vi "SeriellRead-15-07-17.vi"(6 "SkalierungsfaktorHorst":dbl[](array[numeric]), 7 "VorwortHorst":string[](array[string]), 8 "error in":errorcluster, 9 "Zwischenspeicher":string[](array[string]), 10 "Senden?":bool[](array[boolean]), 11 "FPGA VI Reference In":refnum<k20>) -> (1 "Senden?":bool[](array[boolean]), 2 "Zwischenspeicher":string[](array[string]), 3 "error out":errorcluster)   [LabVIEW 2017]
uses:
  GVECDs.vi
  <vilib>/rvi/interface/nirviMethod/nirviMethod.xnode
  FPGA Bitfiles/HAGAR-V_FPGATarget_FPGA-Programm-05_gdVwCsZS6sg.lvbitx
  FPGA/FPGA-Programm-05-17.vi
  <vilib>/FPGAPlugInAG/cRIO-9114/niLvFpga_ReadFifo_cRIO-9114.vi
  <vilib>/rvi/errors/niLvFpgaMergeErrorWithErrorCode.vi
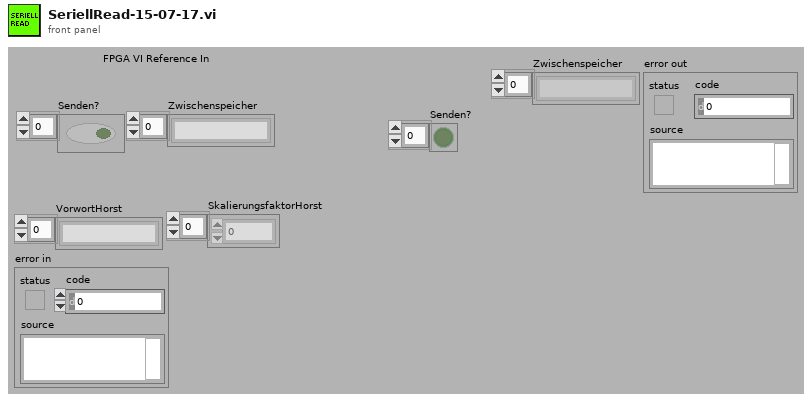
[diagram p1: front panel]
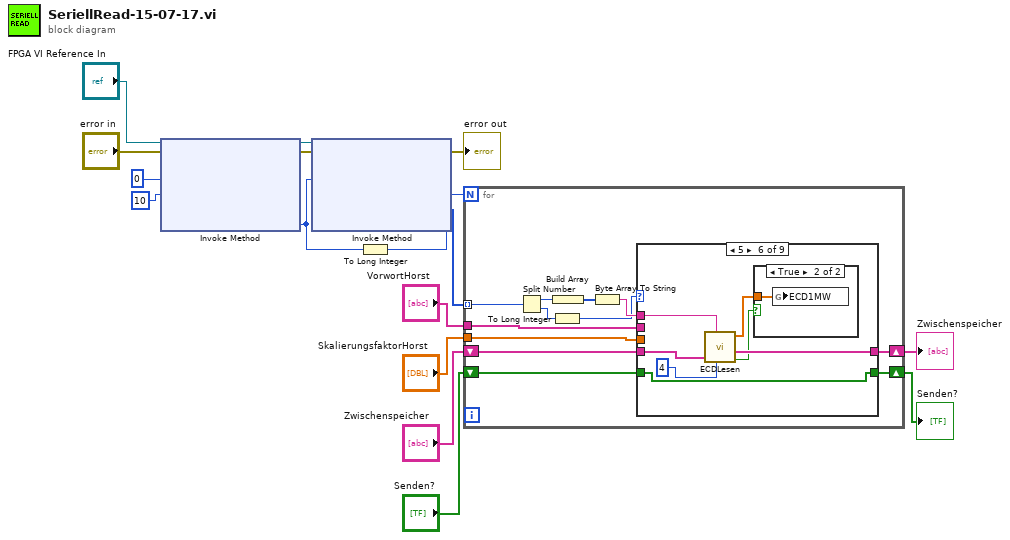
[diagram p0: block diagram]
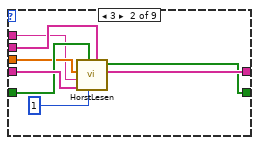
[diagram p3: hidden frame]
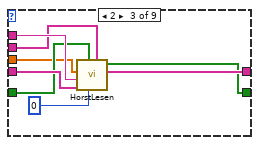
[diagram p4: hidden frame]
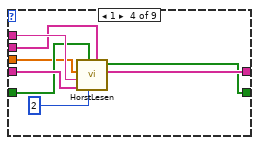
[diagram p5: hidden frame]
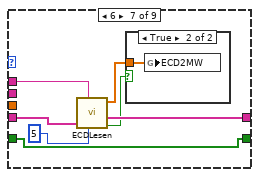
[diagram p8: hidden frame]
diagram:
  n1 = xnode "Invoke Method"("FPGA-VI-Referenz (Eingang)"="FPGA VI Reference In", "Fehler (Eingang)"="error in", "Anzahl der Elemente"=u32 0 ("Number of Elements"), "Timeout (ms)"=10) -> ("FPGA-VI-Referenz (Ausgang)"=w12:refnum<k20>, "Fehler (Ausgang)"=w3:errorcluster, "Verbleibende Elemente"=w15:u32)  [unwired: 1 out]
  n2 = xnode "Invoke Method"("FPGA-VI-Referenz (Eingang)"=w12, "Fehler (Eingang)"=w3, "Anzahl der Elemente"=w15) -> ("Fehler (Ausgang)"=→"error out":errorcluster, "Daten"=w11:u16[])  [unwired: 1 in, 2 out]
  n3 = To Long Integer(number=w15) -> (32bit integer=w16:i32)
  n4 = for {
    N: w16 -> [_]
    tunnel: w11 -> [w28] mode=indexing
    shift-right: [w24] -> w8
    shift-left: "Senden?" -> [w23]
    shift-right: [w25] -> w7
    shift-left: "Zwischenspeicher" -> [w26]
    tunnel: "VorwortHorst" -> [w19]
    tunnel: "SkalierungsfaktorHorst" -> [w18]
    n5 = Split Number(x=w28) -> (hi(x)=w22:u8, lo(x)=w20:u8)
    n6 = To Long Integer(number=w20) -> (32bit integer=w17:i32)
    n7 = Build Array(w22) -> (w21:u8[])
    n8 = Byte Array To String(unsigned byte array=w21) -> (string=w27:string)
    n9 = case shown="5" w17 {
      tunnel: w27 -> [_ w31 w46 w54 _ w63 w71 _ _]
      tunnel: w26 -> [w30 w38 w45 w53 w56 w62 w70 w73 w75]
      tunnel: [w30 w37 w44 w52 w56 w61 w69 w73 w75] -> w25
      tunnel: [w29 w36 w43 w51 w55 w57 w65 w74 w76] -> w24
      tunnel: w23 -> [w29 w35 w42 w50 w55 w57 w65 w74 w76]
      tunnel: w19 -> [_ w34 w41 w49 _ _ _ _ _]
      tunnel: w18 -> [_ w33 w40 w48 _ _ _ _ _]
      frame 0, Default {
      }
      frame 3 {
        n10 = call "HorstLesen.vi"("VorwortHorst"=w34, "Port"=1, "Senden?"=w35, "Zwischenspeicher"=w38, "string"=w31, "SkalierungsfaktorHorst"=w33) -> ("Zwischenspeicher"=w37:string[], "Senden?"=w36:bool[])  [unwired: 4 in]
      }
      frame 2 {
        n11 = call "HorstLesen.vi"("VorwortHorst"=w41, "Port"=0, "Senden?"=w42, "Zwischenspeicher"=w45, "string"=w46, "SkalierungsfaktorHorst"=w40) -> ("Zwischenspeicher"=w44:string[], "Senden?"=w43:bool[])  [unwired: 4 in]
      }
      frame 1 {
        n12 = call "HorstLesen.vi"("VorwortHorst"=w49, "Port"=2, "Senden?"=w50, "Zwischenspeicher"=w53, "string"=w54, "SkalierungsfaktorHorst"=w48) -> ("Zwischenspeicher"=w52:string[], "Senden?"=w51:bool[])  [unwired: 4 in]
      }
      frame 4 {
      }
      frame 5 {
        n13 = call "ECDLesen.vi"("string"=w63, "Zwischenspeicher"=w62, "Port"=4) -> ("ECDMW"=w59:dbl[], "Zwischenspeicher"=w61:string[], "ECDEmpfangen?"=w60:bool)  [unwired: 3 in]
        n14 = case shown="True" w60 {
          tunnel: w59 -> [_ w64]
          frame False {
          }
          frame True {
            n15 = global write "GVECDs.vi" "ECD1MW"(w64) -> ()
          }
        }
      }
      frame 6 {
        n16 = call "ECDLesen.vi"("string"=w71, "Zwischenspeicher"=w70, "Port"=5) -> ("ECDMW"=w67:dbl[], "Zwischenspeicher"=w69:string[], "ECDEmpfangen?"=w68:bool)  [unwired: 3 in]
        n17 = case shown="True" w68 {
          tunnel: w67 -> [_ w72]
          frame False {
          }
          frame True {
            n18 = global write "GVECDs.vi" "ECD2MW"(w72) -> ()
          }
        }
      }
      frame 7 {
      }
      frame 8 {
      }
    }
  }
  "Senden?" <- w8
  "Zwischenspeicher" <- w7
